vi "TestStage2.vi"() -> ()   [LabVIEW 2013]
uses:
  <vilib>/Utility/file.llb/Write To Spreadsheet File (DBL).vi
panel:
  out "iteration":i32
  out "currentPosition":dbl
  in  "Motor COM Port":refnum<visa-resource-name>="COM4"
  in  "Encoder COM Port":refnum<visa-resource-name>="COM1"
  in  "nRuns":i32
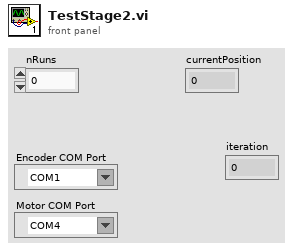
[diagram p1: front panel]
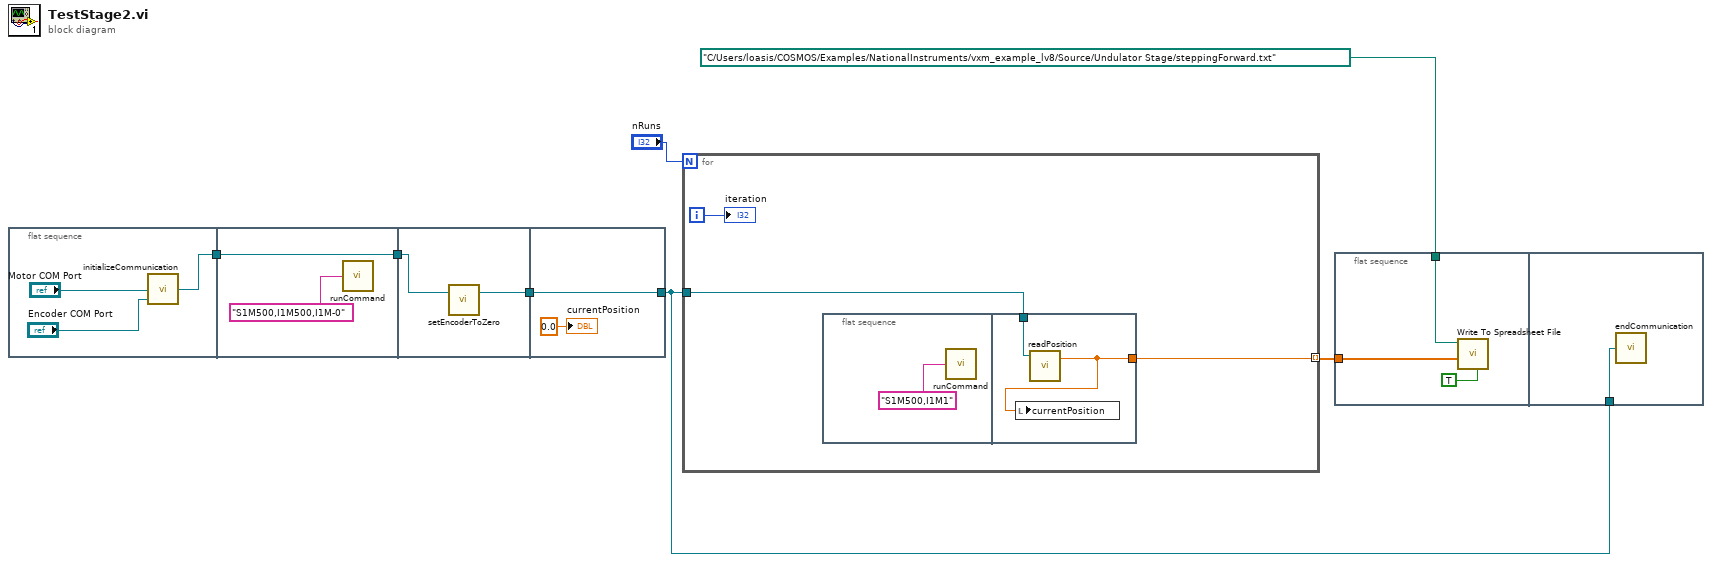
[diagram p0: block diagram]
diagram:
  n1 = flat-sequence {
    tunnel: [w8] -> w7
    tunnel: [w11] -> w6
    tunnel: w7 -> [w11]
    tunnel: w6 -> [w14]
    tunnel: [w13] -> w5
    tunnel: [w16] -> w1
    tunnel: w5 -> [w16]
    frame #0 {
      n2 = call "initializeCommunication.vi"("Encoder COM Port"="Encoder COM Port", "Motor COM Port"="Motor COM Port") -> ("Encoder VISA Resource Name (out)"=w8:refnum<visa-resource-name>)  [unwired: 1 in]
    }
    frame #1 {
      n3 = call "runCommand.vi"("command"="S1M500,I1M500,I1M-0") -> ()  [unwired: 1 in]
    }
    frame #2 {
      n4 = call "setEncoderToZero.vi"("VISA resource name"=w14) -> ("VISA resource name out"=w13:refnum<visa-resource-name>)  [unwired: 1 in, 1 out]
    }
    frame #3 {
      "currentPosition" <- 0.0 ("currentPosition")
    }
  }
  n5 = for {
    N: "nRuns" -> [_]
    tunnel: w1 -> [w19]
    tunnel: [w18] -> w2 mode=indexing
    i -> [w17]
    n6 = flat-sequence {
      tunnel: w19 -> [w22]
      tunnel: [w21] -> w18
      frame #0 {
        n7 = call "runCommand.vi"("command"="S1M500,I1M1") -> ()  [unwired: 1 in]
      }
      frame #1 {
        n8 = call "readPosition.vi"("VISA resource name"=w22) -> ("position"=w21:dbl)  [unwired: 1 in, 2 out]
        n9 = local write "currentPosition"(w21) -> ()
      }
    }
    "iteration" <- w17
  }
  n10 = flat-sequence {
    tunnel: path "C:/Users/loasis/COSMOS/Examples/NationalInstruments/vxm_example_lv8/Source/Undulator Stage/steppingForward.txt" ("file path (dialog if empty)") -> [w25]
    tunnel: w2 -> [w23]
    tunnel: w1 -> [w26]
    frame #0 {
      n11 = call-poly <vilib>:"Write To Spreadsheet File.vi"("transpose? (no:F)"=TRUE, "1D data"=w23, "file path (dialog if empty)"=w25) -> ()  [unwired: 5 in, 1 out]
    }
    frame #1 {
      n12 = call "endCommunication.vi"("Encoder COM Port"=w26) -> ()  [unwired: 1 in]
    }
  }
